vi "Generate Simulated Data.vi"(8 "error in (no error)":T2 caption="entrée d'erreur (pas d'erreur)", 11 "Type de signal":T1) -> (0 "error out":T2 caption="sortie d'erreur", 2 "Données du graphe":waveform(dbl)[](array[waveform]))   [LabVIEW 2020, in "Acquisition.lvlib"]
doc: "Génère des exemples de waveforms en fonction du type de signal dans l'entrée Configuration du matériel."
uses:
  Acquisition.lvlib
  Signal Type.ctl
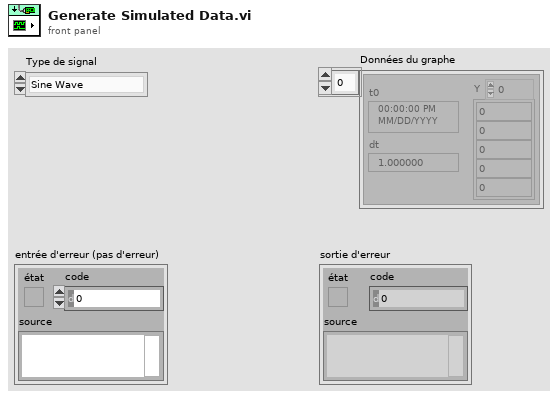
[diagram p1: front panel]
types:
  T1 = typedef "Acquisition.lvlib/Signal Type.ctl" = enum16{"Sine Wave", "Square with Noise", "Signal triangulaire", "Simulation DAQ"}
  T2 = cluster{"état":bool, "code":i32, "source":string}
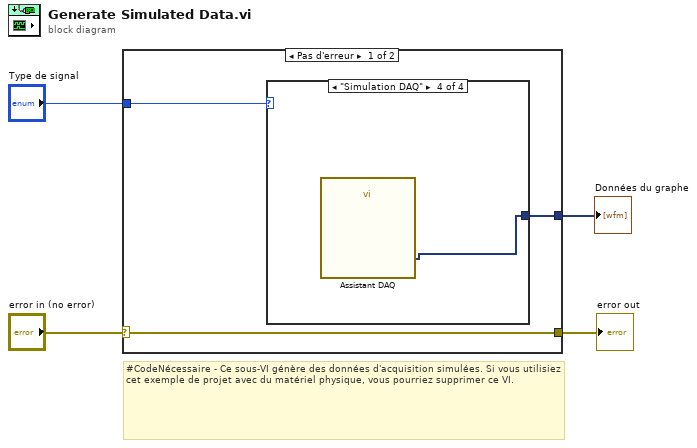
[diagram p0: block diagram]
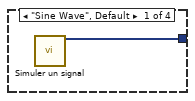
[diagram p2: hidden frame]
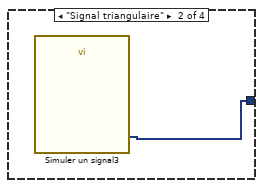
[diagram p3: hidden frame]
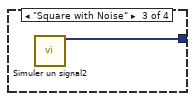
[diagram p4: hidden frame]
diagram:
  # "#CodeNécessaire - Ce sous-VI génère des données d'acquisition simulées. Si vous utilisiez cet exemple de projet avec du matériel physique, vous pourriez supprimer ce VI."
  n1 = case shown="Pas d'erreur" "error in (no error)" {
    selector: "error in (no error)" -> [w7 w12]
    tunnel: [w7 w12] -> w3
    tunnel: [w6 _] -> w2
    tunnel: "Type de signal" -> [w5 _]
    frame No Error {
      n2 = case shown="\"Simulation DAQ\"" w5 {
        tunnel: [w8 w9 w10 w11] -> w6
        frame "Sine Wave", Default {
          n3 = call "Simuler un signal"() -> ("Sine"=w8:dynamicdata)  [unwired: 14 in, 1 out]
        }
        frame "Signal triangulaire" {
          n4 = call "Simuler un signal3"() -> ("Triangle"=w9:dynamicdata)  [unwired: 14 in, 1 out]
        }
        frame "Square with Noise" {
          n5 = call "Simuler un signal2"() -> ("Square with Gaussian Noise"=w10:dynamicdata)  [unwired: 14 in, 1 out]
        }
        frame "Simulation DAQ" {
          n6 = call "Assistant DAQ"() -> ("data"=w11:dynamicdata)  [unwired: 17 in, 2 out]
        }
      }
    }
    frame Error {
    }
  }
  "error out" <- w3
  "Données du graphe" <- w2
